vi "Clase7c.vi"() -> ()   [LabVIEW 2011]
panel:
  out "SUMA150":dbl
  out "CONTADOR":dbl
  out "VELOCIDAD PROMEDIO":dbl
  out "Velocidad":dbl(knob) scale=0.0..220.0
  # "Generar 10 prueba de velocidad luego sumar las velocidades mayores a 150 y \nobtener su promedio"
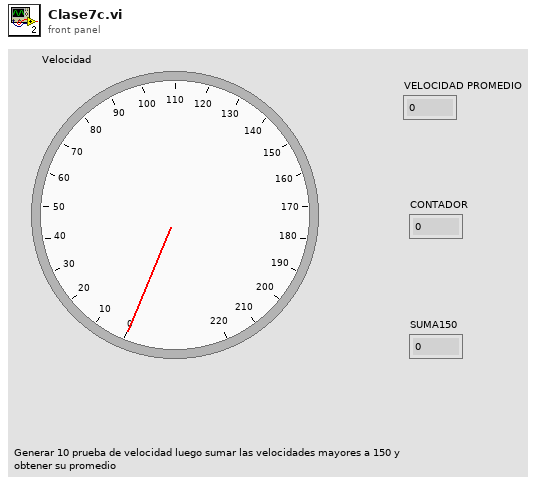
[diagram p1: front panel]
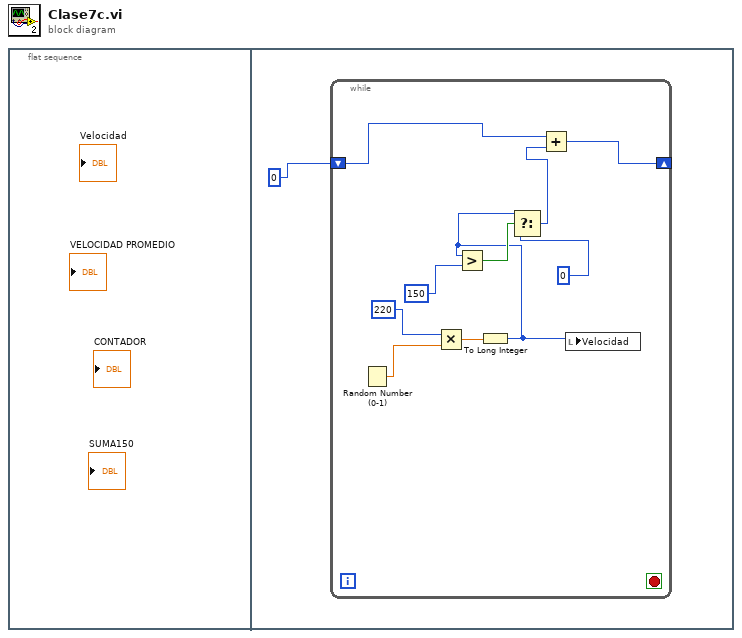
[diagram p0: block diagram]
diagram:
  n1 = flat-sequence {
    frame #0 {
    }
    frame #1 {
      n2 = while {
        shift-right: [w10] -> _
        shift-left: 0 -> [w11]
        stop <- _ stop-if-true
        n3 = Random Number (0-1)() -> (number: 0 to 1=w7:dbl)
        n4 = Multiply(x=220, y=w7) -> (x*y=w6:dbl)
        n5 = To Long Integer(number=w6) -> (32bit integer=w2:i32)
        n6 = Greater?(x=w2, y=150) -> (0:w4:bool)
        n7 = Select(t=w2, s=w4, f=0) -> (s? t:f=w9:i32)
        n8 = Add(x=w11, y=w9) -> (x+y=w10:i32)
        n9 = local write "Velocidad"(w2) -> ()
      }
    }
  }
